vi "uintSubstract.vi"(8 "Error in (no error)":errorcluster, 10 "Uint2 in":refnum<class "UintClass.lvclass">, 11 "Uint1 in":refnum<class "UintClass.lvclass">) -> (0 "Error out":errorcluster, 1 "Timing":u32, 3 "Uint1 + Uint2":refnum<class "UintClass.lvclass">)   [LabVIEW 2011, in "UintClass.lvclass"]
uses:
  UintClass.lvclass
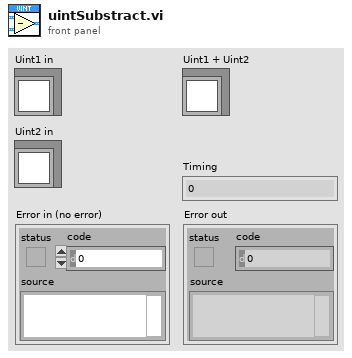
[diagram p1: front panel]
types:
  T1 = typedef "UintClass.lvclass/enumBase.ctl" = u16
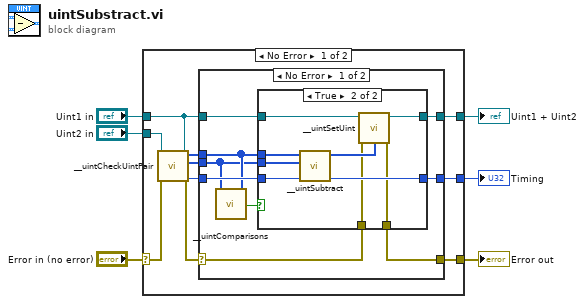
[diagram p0: block diagram]
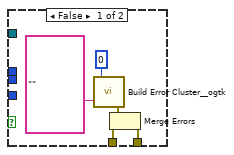
[diagram p2: hidden frame]
diagram:
  n1 = case shown="No Error" "Error in (no error)" {
    selector: "Error in (no error)" -> [w13 w41]
    tunnel: [w11 w41] -> w5
    tunnel: "Uint2 in" -> [w14 _]
    tunnel: "Uint1 in" -> [w7 _]
    tunnel: [w16 _] -> w2
    tunnel: [w15 _] -> w1
    frame No Error {
      n2 = call "__uintCheckUintPair.vi"("Error in (no error)"=w13, "Uint2 in"=w14, "Uint1 in"=w7) -> ("Error out"=w12:errorcluster, "Uint2 out"=w9:u8[], "Uint1 out"=w10:u8[], "Base out"=w8:T1)  [unwired: 5 in]
      n3 = case shown="No Error" w12 {
        selector: w12 -> [w21 w40]
        tunnel: [w25 _] -> w16
        tunnel: [w24 _] -> w15
        tunnel: [w20 w40] -> w11
        tunnel: w10 -> [w19 _]
        tunnel: w9 -> [w18 _]
        tunnel: w8 -> [w23 _]
        tunnel: w7 -> [w22 _]
        frame No Error {
          n4 = call "__uintComparisons.vi"("Uint2 in"=w18, "Uint1 in"=w19) -> ("Uint1 >= Uint2"=w17:bool)  [unwired: 3 in, 6 out]
          n5 = case shown="True" w17 {
            tunnel: [_ w39] -> w25
            tunnel: [_ w37] -> w24
            tunnel: w23 -> [_ w36]
            tunnel: w22 -> [_ w35]
            tunnel: w21 -> [w30 w34]
            tunnel: [w29 w33] -> w20
            tunnel: w19 -> [_ w32]
            tunnel: w18 -> [_ w31]
            frame False {
              n6 = call <userlib>:"Build Error Cluster__ogtk.vi"("String to Prepend to source (\"\")"="" ("String to Prepend to source (\"\")"), "code"=0) -> ("error out"=w28:errorcluster)
              n7 = Merge Errors(w28, w30) -> (w29:errorcluster)
            }
            frame True {
              n8 = call "__uintSubtract.vi"("Base (decimal)"=w36, "Uint2 in"=w31, "Uint1 in"=w32) -> ("Timing substraction"=w39:u32, "Uint1 - Uint2"=w38:u8[])  [unwired: 7 in]
              n9 = call "__uintSetUint.vi"("Error in (no error)"=w34, 10:"Uint in"=w38, 11:"Uint in"=w35) -> ("Error out"=w33:errorcluster, "Uint out"=w37:refnum<class "UintClass.lvclass">)  [unwired: 7 in]
            }
          }
        }
        frame Error {
        }
      }
    }
    frame Error {
    }
  }
  "Error out" <- w5
  "Uint1 + Uint2" <- w1
  "Timing" <- w2
